vi "FileWriteTiming.vi"(8 "Loop counter":i32, 11 "WriteData":bool) -> (2 "Write counter":i32, 3 "Time (s)":dbl)   [LabVIEW 2018]
uses:
  <vilib>/functionblocks/Edge Detection/Edge Detect/Edge Detect.vi
  <vilib>/functionblocks/FB Core/FB Core.xnode
  <vilib>/functionblocks/NI_FunctionBlock Libraries.lvlib
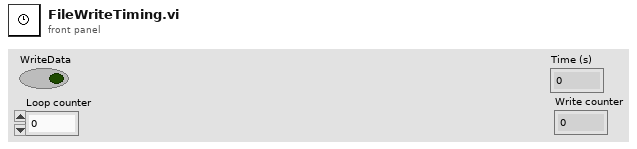
[diagram p1: front panel]
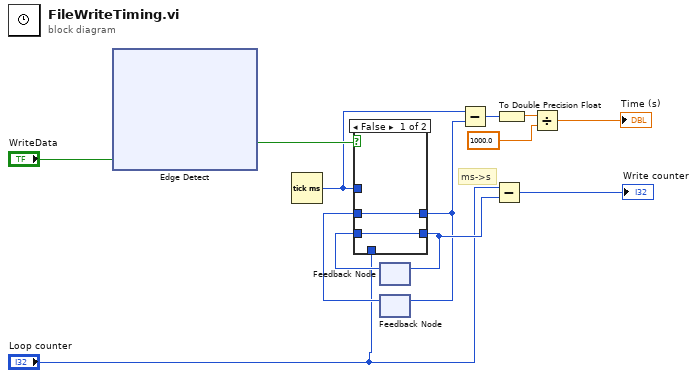
[diagram p0: block diagram]
diagram:
  # "ms->s"
  n1 = xnode "Edge Detect"("input 1"="WriteData") -> ("output"=w13:bool)  [unwired: 2 in, 1 out]
  n2 = Tick Count (ms)() -> (millisecond timer value=w12:u32)
  n3 = feedback #1() -> (w7:i32)  [unwired: 1 in]
  n4 = feedback #2() -> (w5:u32)  [unwired: 1 in]
  n5 = case shown="False" w13 {
    tunnel: w12 -> [_ w17]
    tunnel: [w14 w17] -> w6
    tunnel: "Loop counter" -> [_ w16]
    tunnel: [w15 w16] -> w8
    tunnel: w7 -> [w15 _]
    tunnel: w5 -> [w14 _]
    frame False {
    }
    frame True {
    }
  }
  n6 = feedback-in #1(w8) -> ()
  n7 = feedback-in #2(w6) -> ()
  n8 = Subtract(x=w12, y=w6) -> (x-y=w11:u32)
  n9 = Subtract(x="Loop counter", y=w8) -> (x-y=→"Write counter":i32)
  n10 = To Double Precision Float(number=w11) -> (double precision float=w10:dbl)
  n11 = Divide(x=w10, y=1000.0) -> (x/y=→"Time (s)":dbl)
